vi "QueryServer_SetTestDataTypesResults.vi"(6 "error in (no error)":errorcluster, 8 "TestDataTypesParameters":T1, 9 "gRPCid":T3) -> (0 "error out":errorcluster, 3 "gRPCid out":T3)   [LabVIEW 2019, in "labview-grpc-query-server.lvlib"]
uses:
  labview-grpc-query-server.lvlib
  VIs/grpcId.ctl
  QueryServer_TestDataTypesParameters.ctl
  QueryServer_DataTypeTest.ctl
  build/Debug/labview_grpc_server.dll
  VIs/gprc-support.lvlib
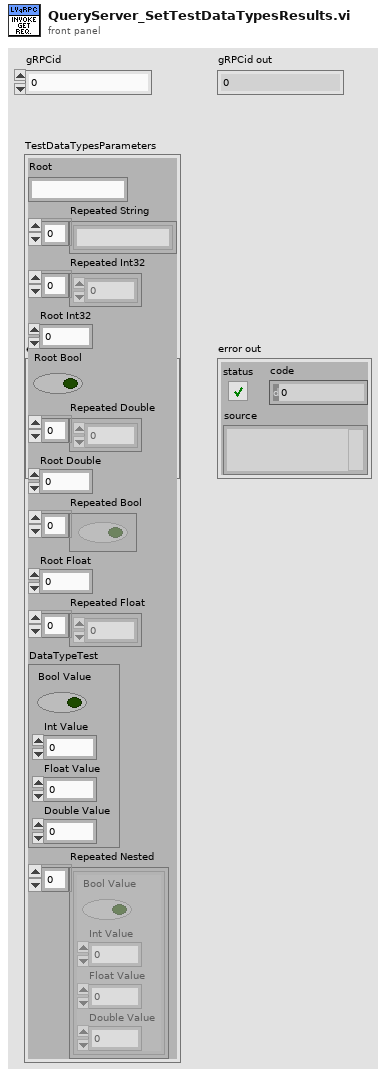
[diagram p1: front panel]
types:
  T1 = typedef "labview-grpc-query-server.lvlib/QueryServer_TestDataTypesParameters.ctl" = cluster{"Root":string, "Repeated String":string[], "Repeated Int32":i32[], "Root Int32":i32, "Root Bool":bool, "Repeated Double":dbl[], "Root Double":dbl, "Repeated Bool":bool[], "Root Float":sgl, "Repeated Float":sgl[], "DataTypeTest":T2, "Repeated Nested":T2[]}
  T2 = typedef "labview-grpc-query-server.lvlib/QueryServer_DataTypeTest.ctl" = cluster{"Bool Value":bool, "Int Value":i32, "Float Value":sgl, "Double Value":dbl}
  T3 = typedef "gprc-support.lvlib/grpcId.ctl" = u64
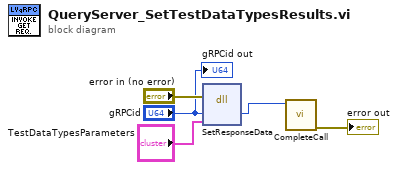
[diagram p0: block diagram]
diagram:
  n1 = dll-call lib="C:/dev/labview-grpc-server/build/Debug/labview_grpc_server.dll" fn="SetResponseData"(error in="error in (no error)", "id"="gRPCid", "data"="TestDataTypesParameters") -> ("id"=w2:T3)  [unwired: 4 in, 2 out]
  n2 = call "CompleteCall.vi"("gRPCid"=w2) -> ("error out"=→"error out":errorcluster)  [unwired: 9 in]
  "gRPCid out" <- "gRPCid"
